vi "Add Start Condition.vi"(8 "error in (no error)":errorcluster, 10 "Action":T1, 11 "I2C waveform info":T2) -> (0 "error out":errorcluster, 3 "I2C waveform info out":T2)   [LabVIEW 2009, in "IDW.lvlib"]
doc: "Adds a Start (S) or Repeated Start (Sr) condition to the I2C waveform. \n\nTiming parameters that affect this waveform segment's length are: <b>tSU;DAT</b> (Sr only), <b>tSU;STA</b> (Sr only), <b>tHD;STA </b>, and <b>tHD;DAT</b>"
uses:
  IDW.lvlib
  _Typedefs/Waveform info.ctl
  _Typedefs/Timing - ticks.ctl
  _Typedefs/Default transition action.ctl
  _Typedefs/Bit type.ctl
  _Typedefs/Start action.ctl
  _Private/Polymorphics/Change Bit Value - Single.vi
  _Typedefs/Channel Ring.ctl
  _Private/Polymorphics/Change Bit Value - Multi.vi
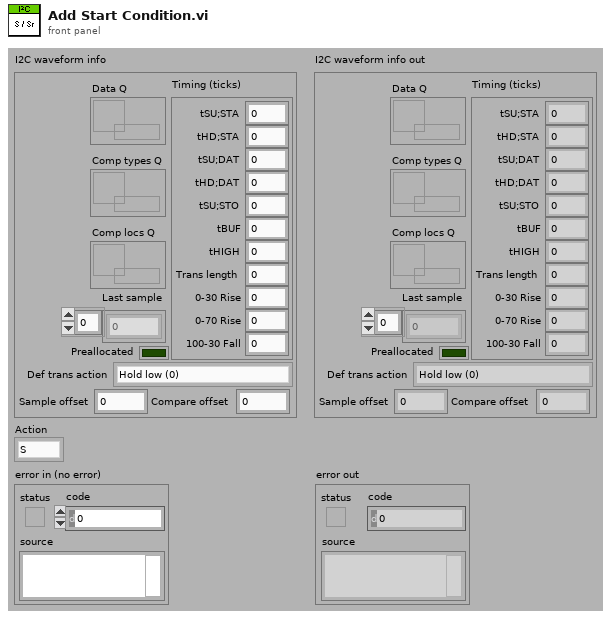
[diagram p1: front panel]
types:
  T1 = typedef "IDW.lvlib/Start action.ctl" = enum16{"S", "Sr"}
  T2 = typedef "IDW.lvlib/Waveform info.ctl" = cluster{"Last sample":u8[], "Sample offset":u64, "Compare offset":u64, "Timing (ticks)":T3, "Preallocated":bool, "Def trans action":T4, "Data Q":refnum<queue>, "Comp types Q":refnum<queue>, "Comp locs Q":refnum<queue>}
  T3 = typedef "IDW.lvlib/Timing - ticks.ctl" = cluster{"tSU;STA":i32, "tHD;STA":i32, "tSU;DAT":i32, "tHD;DAT":i32, "tSU;STO":i32, "tBUF":i32, "tHIGH":i32, "Trans length":i32, "0-30 Rise":i32, "0-70 Rise":i32, "100-30 Fall":i32}
  T4 = typedef "IDW.lvlib/Default transition action.ctl" = enum16{"Hold low (0)", "Release (Z)", "Set up next value", "Hold previous value", "Preserve tHD;DAT and tSU;DAT"}
  T5 = typedef "IDW.lvlib/Channel Ring.ctl" = u16
  T6 = typedef "IDW.lvlib/Channel ring.ctl" = u16
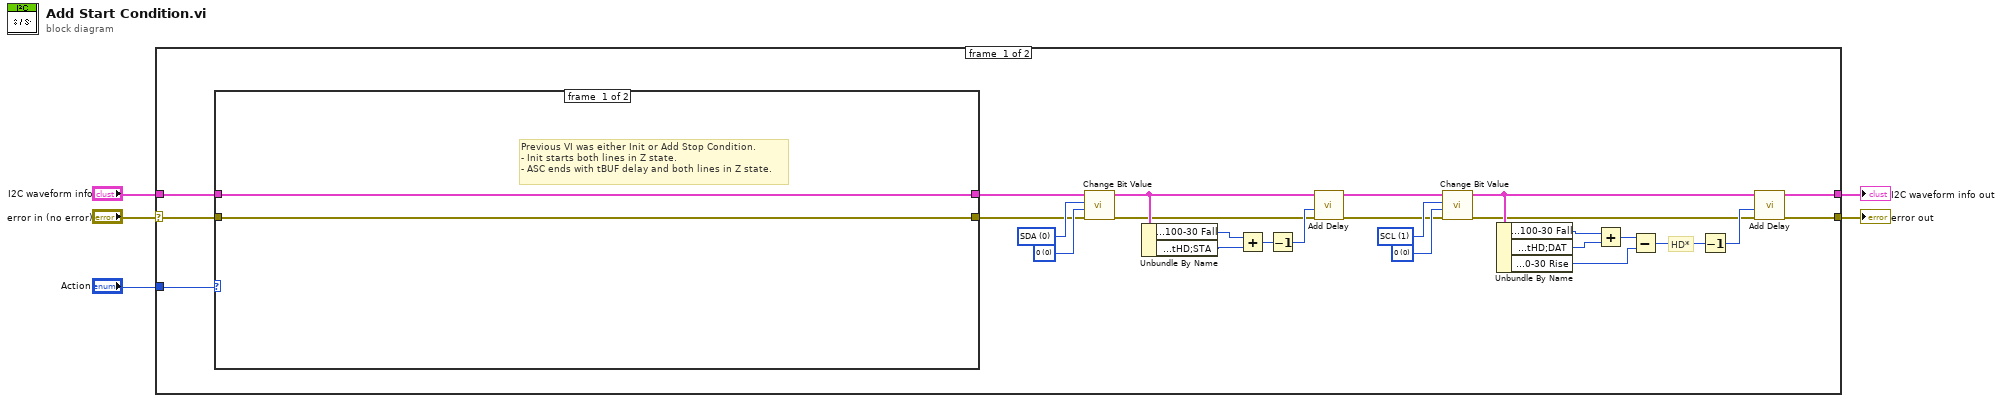
[diagram p0: block diagram]
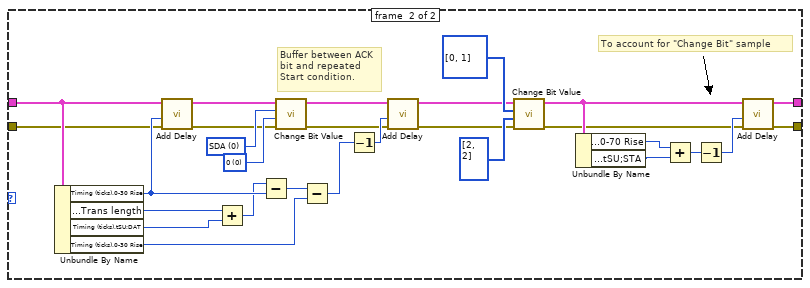
[diagram p2: hidden frame]
diagram:
  n1 = case shown="No Error" "error in (no error)" {
    selector: "error in (no error)" -> [w7 w64]
    tunnel: [w12 w63] -> w5
    tunnel: "Action" -> [w27 _]
    tunnel: "I2C waveform info" -> [w26 w63]
    tunnel: [w6 w64] -> w1
    frame #0 {
      w30 = u8 0 items=["0", "1", "Z", "L", "H", "X", "T", "V"] ("State")
      w29 = T5 1 items=["SDA", "SCL"] ("I2C Ring")
      w31 = u8 0 items=["0", "1", "Z", "L", "H", "X", "T", "V"] ("State")
      w32 = T5 0 items=["SDA", "SCL"] ("I2C Ring")
      # "HD*"
      n2 = case shown="\"Sr\"" w27 {
        tunnel: [w34 w41] -> w23
        tunnel: w26 -> [w34 w51]
        tunnel: [w33 w36] -> w11
        tunnel: w7 -> [w33 w35]
        frame #0 {
          # "Previous VI was either Init or Add Stop Condition.\n- Init starts both lines in Z state.\n- ASC ends with tBUF delay and both lines in Z state."
        }
        frame #1 {
          w58 = u8 0 items=["0", "1", "Z", "L", "H", "X", "T", "V"] ("State")
          w59 = T5 0 items=["SDA", "SCL"] ("I2C Ring")
          w62 = T6[] [0, 1] items=["SDA", "SCL"] ("Bits")
          w61 = u8[] [2, 2] items=["0", "1", "Z", "L", "H", "X", "T", "V"] ("States")
          # "To account for \"Change Bit\" sample"
          # "Buffer between ACK bit and repeated Start condition."
          n3 = Unbundle By Name(w51) -> ("Timing (ticks).0-30 Rise"=w53:i32, "Timing (ticks).Trans length"=w50:i32, "Timing (ticks).tSU;DAT"=w49:i32, "Timing (ticks).0-30 Rise"=w52:i32)
          n4 = call "Add Delay.vi"("error in (no error)"=w35, "# Samples"=w53, "I2C waveform info"=w51) -> ("error out"=w40:errorcluster, "I2C waveform info out"=w56:T2)  [unwired: 1 in, 6 out]
          n5 = Add(x=w50, y=w49) -> (x+y=w48:i32)
          n6 = Subtract(x=w48, y=w53) -> (x-y=w55:i32)
          n7 = call-poly "Change Bit Value.vi"("error in (no error)"=w40, "State"=w58, "Bit"=w59, "I2C waveform info"=w56) -> ("error out"=w39:errorcluster, "I2C waveform info out"=w60:T2)  [unwired: 6 out]
          n8 = Subtract(x=w55, y=w52) -> (x-y=w54:i32)
          n9 = Decrement(x=w54) -> (x-1=w57:i32)
          n10 = call "Add Delay.vi"("error in (no error)"=w39, "# Samples"=w57, "I2C waveform info"=w60) -> ("error out"=w38:errorcluster, "I2C waveform info out"=w47:T2)  [unwired: 1 in, 6 out]
          n11 = call-poly "Change Bit Value.vi"("error in (no error)"=w38, "States"=w61, "Bits"=w62, "I2C waveform info"=w47) -> ("error out"=w37:errorcluster, "I2C waveform info out"=w45:T2)  [unwired: 6 out]
          n12 = Unbundle By Name(w45) -> ("Timing (ticks).0-70 Rise"=w44:i32, "Timing (ticks).tSU;STA"=w43:i32)
          n13 = Add(x=w44, y=w43) -> (x+y=w42:i32)
          n14 = Decrement(x=w42) -> (x-1=w46:i32)
          n15 = call "Add Delay.vi"("error in (no error)"=w37, "# Samples"=w46, "I2C waveform info"=w45) -> ("error out"=w36:errorcluster, "I2C waveform info out"=w41:T2)  [unwired: 1 in, 6 out]
        }
      }
      n16 = call-poly "Change Bit Value.vi"("error in (no error)"=w11, "State"=w31, "Bit"=w32, "I2C waveform info"=w23) -> ("error out"=w10:errorcluster, "I2C waveform info out"=w25:T2)  [unwired: 6 out]
      n17 = Unbundle By Name(w25) -> ("Timing (ticks).100-30 Fall"=w21:i32, "Timing (ticks).tHD;STA"=w22:i32)
      n18 = Add(x=w21, y=w22) -> (x+y=w20:i32)
      n19 = Decrement(x=w20) -> (x-1=w24:i32)
      n20 = call "Add Delay.vi"("error in (no error)"=w10, "# Samples"=w24, "I2C waveform info"=w25) -> ("error out"=w8:errorcluster, "I2C waveform info out"=w28:T2)  [unwired: 1 in, 6 out]
      n21 = call-poly "Change Bit Value.vi"("error in (no error)"=w8, "State"=w30, "Bit"=w29, "I2C waveform info"=w28) -> ("error out"=w9:errorcluster, "I2C waveform info out"=w13:T2)  [unwired: 6 out]
      n22 = Unbundle By Name(w13) -> ("Timing (ticks).100-30 Fall"=w18:i32, "Timing (ticks).tHD;DAT"=w17:i32, "Timing (ticks).0-30 Rise"=w15:i32)
      n23 = Add(x=w18, y=w17) -> (x+y=w16:i32)
      n24 = Subtract(x=w16, y=w15) -> (x-y=w14:i32)
      n25 = Decrement(x=w14) -> (x-1=w19:i32)
      n26 = call "Add Delay.vi"("error in (no error)"=w9, "# Samples"=w19, "I2C waveform info"=w13) -> ("error out"=w6:errorcluster, "I2C waveform info out"=w12:T2)  [unwired: 1 in, 6 out]
    }
    frame #1 {
    }
  }
  "I2C waveform info out" <- w5
  "error out" <- w1
